vi "DO Configuration to Channel Settings.vi"(8 "error in":errorcluster, 9 "default values":dbl[](array[numeric]), 10 "names":string[](array[string]), 11 "digital output mode in":refnum<class "Digital Output Mode.lvclass">) -> (0 "error out":errorcluster, 2 "channel settings":T1[](array[typedef]), 3 "digital output mode out":refnum<class "Digital Output Mode.lvclass">)   [LabVIEW 2017, in "Scan Engine Scripting.lvlib" / "Digital Output Mode.lvclass"]
uses:
  Digital Output Mode.lvclass
  Controls/digital channel settings.ctl
  Scan Engine Scripting.lvlib
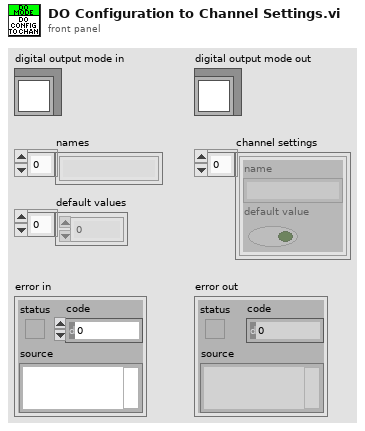
[diagram p1: front panel]
types:
  T1 = typedef "Scan Engine Scripting.lvlib/digital channel settings.ctl" = cluster{"name":string, "default value":bool}
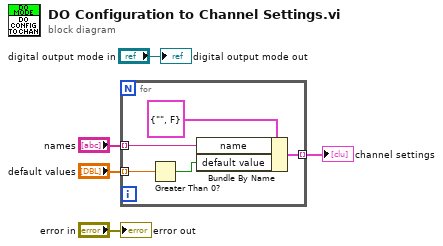
[diagram p0: block diagram]
diagram:
  n1 = for {
    tunnel: "names" -> [w9] mode=indexing
    tunnel: "default values" -> [w8] mode=indexing
    tunnel: [w6] -> w3 mode=indexing
    n2 = Greater Than 0?(x=w8) -> (x > 0?=w7:bool)
    n3 = Bundle By Name(cluster=T1 {"name"="", "default value"=FALSE} ("channel settings"), "name"=w9, "default value"=w7) -> (w6:T1)
  }
  "channel settings" <- w3
  "error out" <- "error in"
  "digital output mode out" <- "digital output mode in"
